vi "Setup Task.vi"(8 "error in":errorcluster, 11 "4300 in":refnum<class "4300.lvclass">) -> (0 "error out":errorcluster, 3 "4300 out":refnum<class "4300.lvclass">)   [LabVIEW 2019, in "4300.lvlib" / "4300.lvclass"]
doc: "This routine sets up the analog acquisition task without any timing characteristics. \nYou must call a finite or continuous task after this call"
uses:
  Library/4300.lvclass
  Library/4300.lvclass/4300.ctl
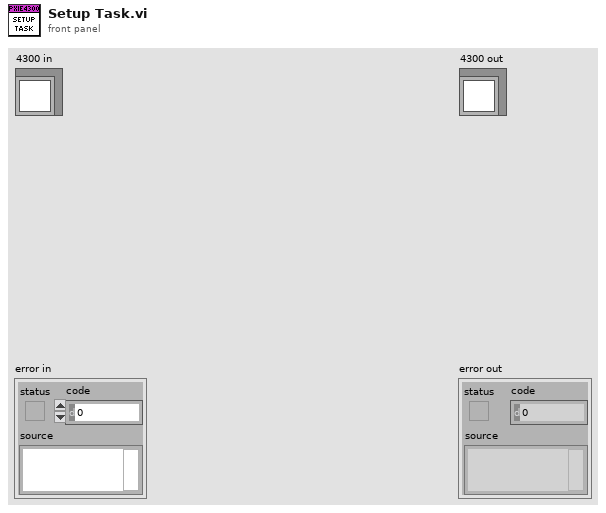
[diagram p1: front panel]
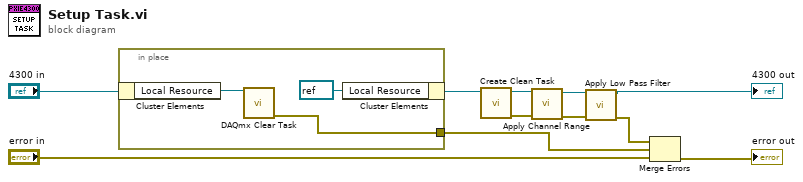
[diagram p0: block diagram]
diagram:
  n1 = in-place {
    in-place-border: [w12] -> w3
    n2 = in-place-cluster #1("4300 in") -> ("Local Resource"=w14:refnum<k21>)
    n3 = call <vilib>:"DAQmx Clear Task.vi"("task in"=w14) -> ("error out"=w12:errorcluster)  [unwired: 14 in]
    n4 = in-place-cluster #1("Local Resource"=refnum<k21> refnum) -> (w11:refnum<class "4300.lvclass">)
  }
  n5 = call "Create Clean Task.vi"("4300 in"=w11) -> ("error out"=w8:errorcluster, "4300 out"=w10:refnum<class "4300.lvclass">)  [unwired: 9 in]
  n6 = call "Apply Channel Range.vi"("error in"=w8, "4300 in"=w10) -> ("error out"=w7:errorcluster, "4300 out"=w9:refnum<class "4300.lvclass">)  [unwired: 8 in]
  n7 = call "Apply Low Pass Filter.vi"("error in"=w7, "4300 in"=w9) -> ("error out"=w4:errorcluster, "4300 out"=→"4300 out":refnum<class "4300.lvclass">)  [unwired: 8 in]
  n8 = Merge Errors(w4, w3, "error in") -> (→"error out":errorcluster)
